vi "Status To Glyph.vi"(3 "Status":T1) -> (1 "Listbox Symbol Ring Constant":i32)   [LabVIEW 2020, in "Result Model.lvclass"]
uses:
  Result Model.lvclass
  Result/Status.ctl
  Result/Result.lvlib
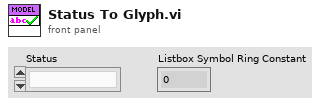
[diagram p1: front panel]
types:
  T1 = typedef "Result.lvlib/Status.ctl" = enum16{"", "Passed", "Failed", "Error", "Skipped", "Setup Error", "Broken", "Teardown Error"}
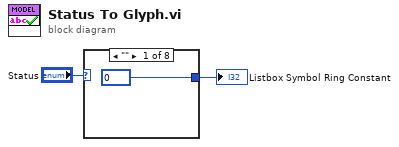
[diagram p0: block diagram]
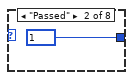
[diagram p2: hidden frame]
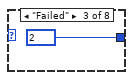
[diagram p3: hidden frame]
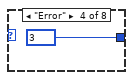
[diagram p4: hidden frame]
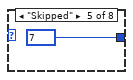
[diagram p5: hidden frame]
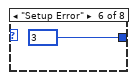
[diagram p6: hidden frame]
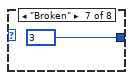
[diagram p7: hidden frame]
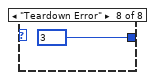
[diagram p8: hidden frame]
diagram:
  n1 = case shown="\"\"" "Status" {
    tunnel: [0 ("Listbox Symbol Ring Constant") 1 ("Listbox Symbol Ring Constant") 2 ("Listbox Symbol Ring Constant") 3 ("Listbox Symbol Ring Constant") 7 ("Listbox Symbol Ring Constant") 3 ("Listbox Symbol Ring Constant") 3 ("Listbox Symbol Ring Constant") 3 ("Listbox Symbol Ring Constant")] -> w1
    frame "" {
    }
    frame "Passed" {
    }
    frame "Failed" {
    }
    frame "Error" {
    }
    frame "Skipped" {
    }
    frame "Setup Error" {
    }
    frame "Broken" {
    }
    frame "Teardown Error" {
    }
  }
  "Listbox Symbol Ring Constant" <- w1
